vi "rpr -- construct operator matrices.vi"() -> ()   [LabVIEW 2010]
panel:
  out "symmetry indexes":i32[](array[numeric])=[556, 646, 974, 1127, 1207, 1578, 1759, 1872, 1895, 2004, 2216, 2256, 2345]
  in  "symmetry blocks":string[][](array[string])
  out "all peaks":i32[](array[numeric])=[556, 646, 974, 1127, 1207, 1578, 1759, 1872, 1895, 2004, 2216, 2256, 2345]
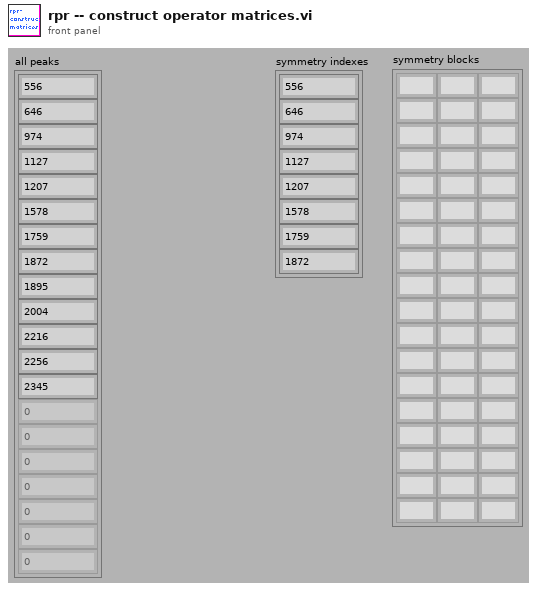
[diagram p1: front panel]
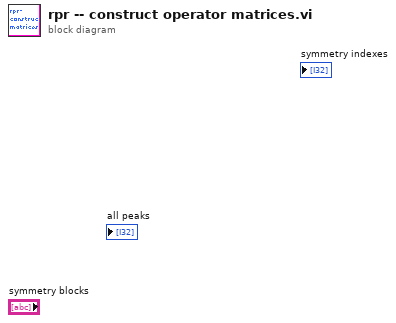
[diagram p0: block diagram]
diagram:
